vi "ReceiveMessages.vi"(6 "timeout(1000)":i32=1000, 8 "error in (no error)":errorcluster, 9 "priority action":string, 10 "default action":string, 11 "Qbus in":refnum<class "Qbus.lvclass">) -> (0 "error out":errorcluster, 1 "message value":variant, 2 "action":string, 3 "Qbus out":refnum<class "Qbus.lvclass">, 4 "exit":bool)   [LabVIEW 2017, in "CmsFpgaBitfileManager.lvlib"]
uses:
  <vilib>/addons/InsightCM/Devices/Shared/Cms/CmsFpgaBitfileManager/CmsFpgaBitfileManager.lvlib
  <vilib>/addons/Qbus/Qbus.lvclass
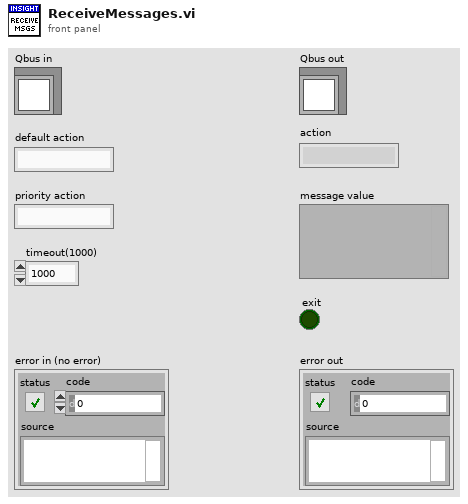
[diagram p1: front panel]
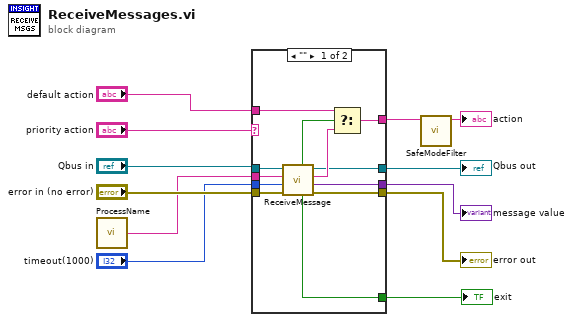
[diagram p0: block diagram]
diagram:
  n1 = call <vilib>:"ProcessName.vi"() -> ("process name"=w1:string)  [unwired: 5 in]
  n2 = case shown="\"\"" "priority action" {
    selector: "priority action" -> [_ w25]
    tunnel: "error in (no error)" -> [w15 w27]
    tunnel: [w21 w27] -> w6
    tunnel: [w20 _] -> w8
    tunnel: [w16 _] -> w3
    tunnel: "default action" -> [w24 _]
    tunnel: [w23 w25] -> w12
    tunnel: [w18 w26] -> w7
    tunnel: "timeout(1000)" -> [w14 _]
    tunnel: "Qbus in" -> [w17 w26]
    tunnel: w1 -> [w13 _]
    frame "" {
      n3 = call <vilib>:"ReceiveMessage.vi"("error in (no error)"=w15, "timeout (0)"=w14, "process name"=w13, "Qbus in"=w17) -> ("error in (no error)"=w21:errorcluster, "message value"=w20:variant, "message name"=w19:string, "Qbus out"=w18:refnum<class "Qbus.lvclass">, "exit"=w16:bool, "timed out"=w22:bool)  [unwired: 2 in]
      n4 = Select(t=w24, s=w22, f=w19) -> (s? t:f=w23:string)
    }
    frame Default {
    }
  }
  "message value" <- w8
  "Qbus out" <- w7
  "error out" <- w6
  "exit" <- w3
  n5 = call <vilib>:"SafeModeFilter.vi"("action in"=w12) -> ("action out"=→"action":string)  [unwired: 10 in]
